vi "sub_UIupdate_rt.vi"(11 "log data":T1) -> (0 "error out":errorcluster)   [LabVIEW 2016]
uses:
  ctl/log_data.ctl
  ctl/UI_cmd-ctl.ctl
  <vilib>/Analysis/baseanly.llb/Mean (DBL).vi
  Global.vi
  <vilib>/Analysis/baseanly.llb/Unimode.vi
  <vilib>/Analysis/NI_AALBase.lvlib
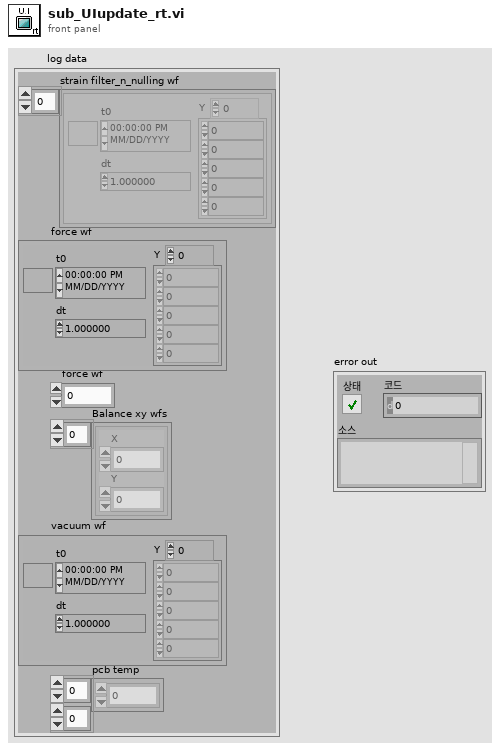
[diagram p1: front panel]
types:
  T1 = typedef "log_data.ctl" = cluster{"strain filter_n_nulling wf":waveform(dbl)[], "force wf":waveform(dbl), "force":dbl, "Balance xy wfs":cluster{"X":dbl, "Y":dbl}[], "vacuum kpa wf":waveform(dbl), "pcb temp":dbl[][]}
  T2 = typedef "UI_cmd-ctl.ctl" = enum16{"default", "create", "read"}
  T3 = typedef "UI_ctl.ctl" = cluster{"Heater temp":refnum<vi>, "Heater chart":refnum<vi>, "vacuum (kpa)":refnum<vi>, "Balance xy graph":refnum<vi>, "Strain chart w cal":refnum<vi>, "Pickup force":refnum<vi>, "Pickup time":refnum<vi>, "Force chart":refnum<vi>, "Force graph T":refnum<vi>, "vacuum chart":refnum<vi>, "vacuum rt":refnum<vi>, "Strain raw graph":refnum<vi>, "Strain raw chart":refnum<vi>, "Bonding time":refnum<vi>, "Bonding force":refnum<vi>, "Balance":refnum<vi>, "Filtered force graph":refnum<vi>, "ROI intensity":refnum<vi>, "Heater_rt":refnum<vi>, "Detach force":refnum<vi>, "Force rt":refnum<vi>, "Mixed signal":refnum<vi>}
  T4 = typedef "config_ctl.ctl" = cluster{"Lower Cut-Off":dbl, "Vacuum Trigger level":dbl, "state settings":cluster{"method":enum32{"histogram", "peak", "auto select"}, "histogram size":i32, "histogram method":enum16{"mode"}, "reserved":dbl}, "SPA-300 Setting":cluster{"Bonding force (g)":dbl, "Bonding time (ms)":dbl, "Pickup force (g)":dbl, "Pickup time (ms)":dbl, "Speed":enum16{"Slow", "Fast"}}, "sensor file":path}
  T5 = cluster{"PCB temp":refnum<vi>, "Vacuum":refnum<vi>, "PCB config":refnum<vi>, "Balance_x":refnum<vi>, "Balance_y":refnum<vi>}
  T6 = typedef "data.ctl" = cluster{"Bonding force":dbl, "Bonding time":dbl, "Bonding index":dbl, "Pickup force":dbl, "Pickup time":dbl, "Pickup index":dbl, "Detach force":dbl, "Detach time":dbl, "Detach index":dbl, "Heater temp rt":dbl, "Vacuum rt":dbl, "IR raw data":i16[][], "IR temp data":dbl[][], "vacuum raw wf":waveform(dbl), "vacuum kpa wf":waveform(dbl), "strain raw wf":waveform(dbl)[], "Force rt":dbl, "Vacuum T":dbl, "Heater temp T":dbl, "Balance xy arrays":cluster{dbl, dbl}[], "Balance xy":cluster{dbl, dbl}[], "Bonding wf index":dbl, "Pickup wf index":dbl, "Bonding rising index":dbl, "Bonding falling index":dbl, "Pickup rising index":dbl, "Pickup falling index":dbl}
  T7 = cluster{"Force rt":dbl, "Vacuum rt":dbl, "Heater temp rt":dbl}
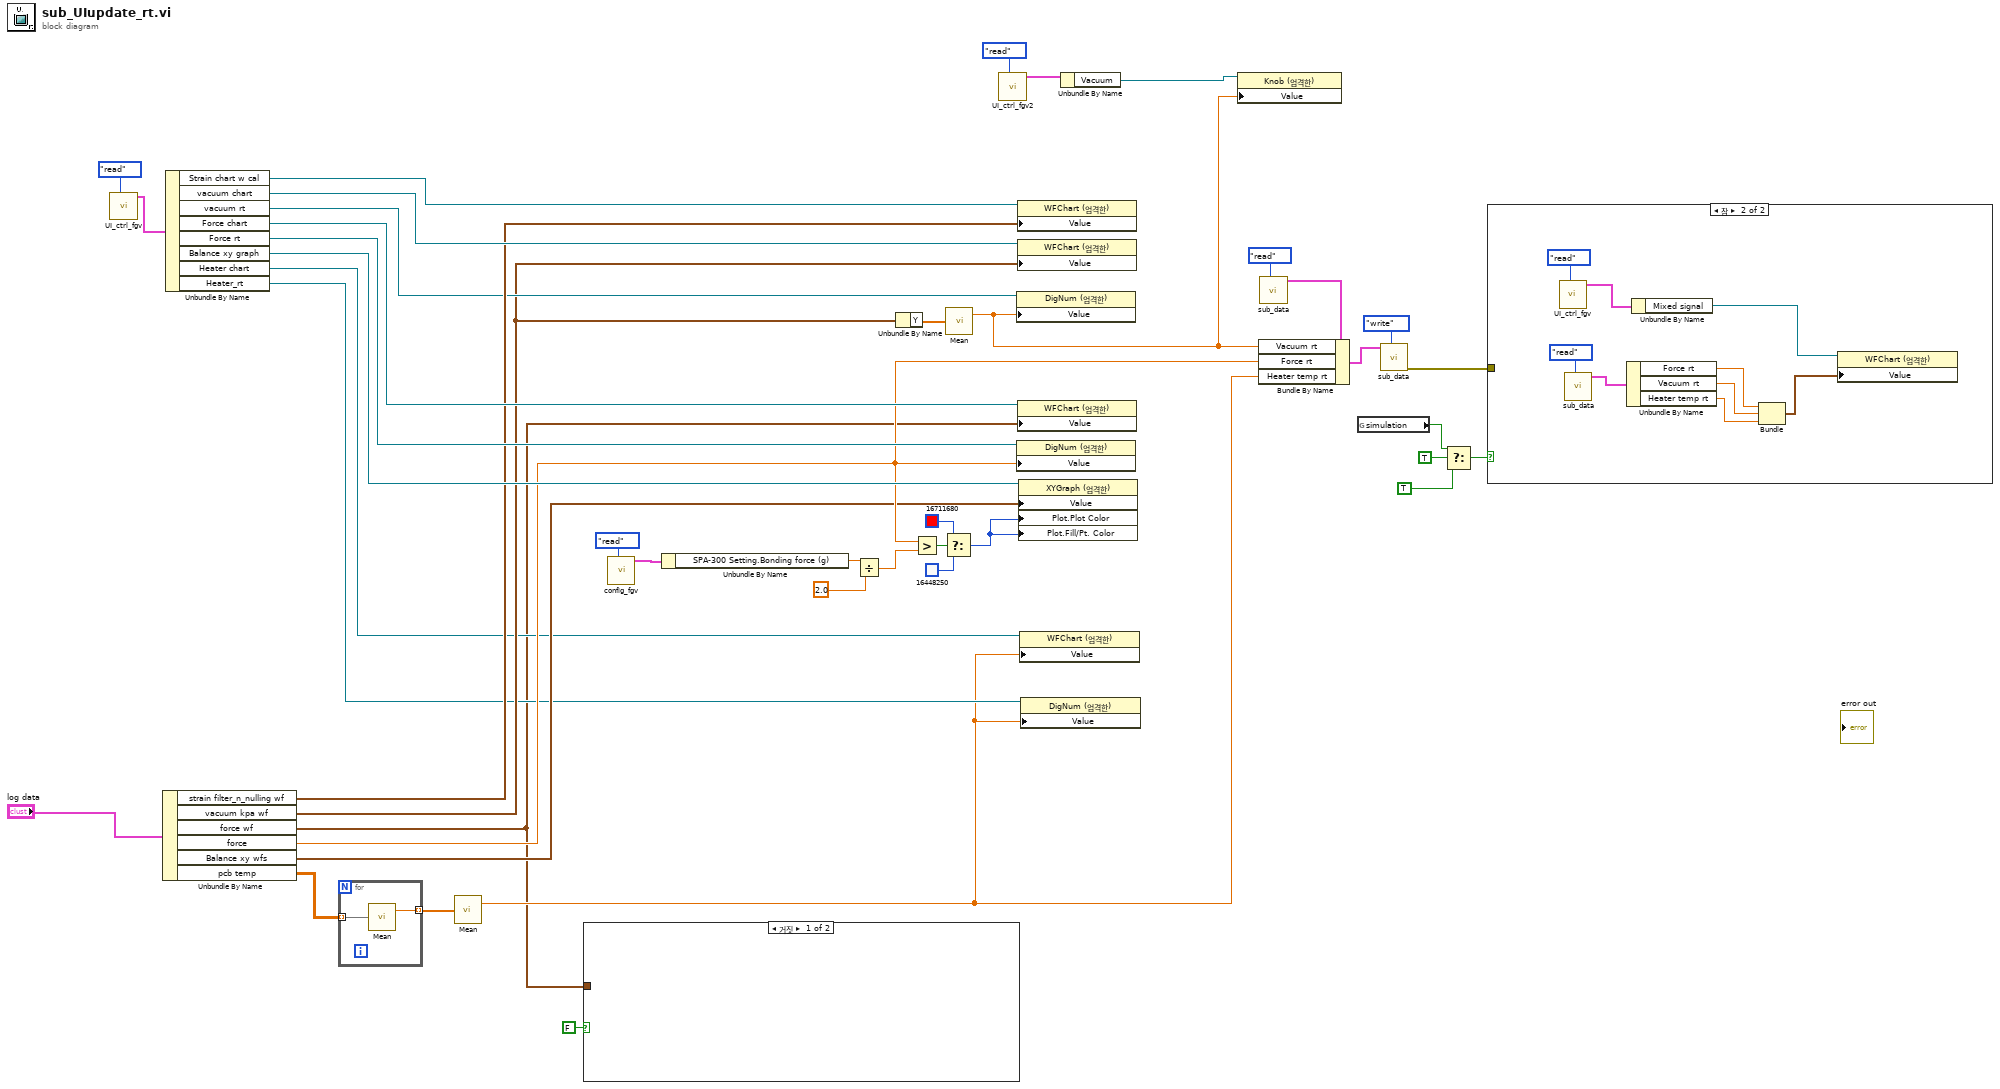
[diagram p0: block diagram]
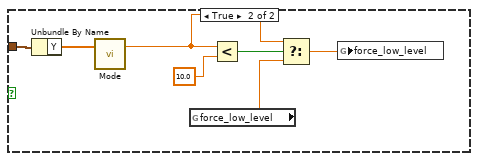
[diagram p2: hidden frame]
diagram:
  n1 = call "UI_ctrl_fgv.vi"("cmd"=UI_cmd-ctl."read") -> ("UI cluster out"=w39:T3)  [unwired: 10 in]
  n2 = Unbundle By Name("log data") -> ("strain filter_n_nulling wf"=w36:waveform(dbl)[], "vacuum kpa wf"=w31:waveform(dbl), "force wf"=w1:waveform(dbl), "force"=w19:dbl, "Balance xy wfs"=w14:cluster{"X":dbl, "Y":dbl}[], "pcb temp"=w18:dbl[][])
  n3 = Unbundle By Name(w39) -> ("Strain chart w cal"=w37:refnum<vi>, "vacuum chart"=w38:refnum<vi>, "vacuum rt"=w34:refnum<vi>, "Force chart"=w41:refnum<vi>, "Force rt"=w42:refnum<vi>, "Balance xy graph"=w43:refnum<vi>, "Heater chart"=w13:refnum<vi>, "Heater_rt"=w12:refnum<vi>)
  n4 = for {
    tunnel: w18 -> [w45] mode=indexing
    tunnel: [w44] -> w17 mode=indexing
    n5 = call-poly <vilib>:"Mean.vi"("X"=w45) -> ("mean"=w44:dbl)  [unwired: 1 out]
  }
  n6 = call-poly <vilib>:"Mean.vi"("X"=w17) -> ("mean"=w11:dbl)  [unwired: 1 out]
  n7 = case shown="거짓" FALSE {
    tunnel: w1 -> [_ w52]
    frame False {
    }
    frame True {
      n8 = Unbundle By Name(w52) -> ("Y"=w51:dbl[])
      n9 = call-poly <vilib>:"Mode.vi"("X"=w51) -> ("mode"=w48:dbl)  [unwired: 1 in, 1 out]
      n10 = global read "Global.vi" "force_low_level"() -> (w47:dbl)
      n11 = Less?(x=w48, y=10.0) -> (x < y?=w49:bool)
      n12 = Select(t=w48, s=w49, f=w47) -> (s? t:f=w46:dbl)
      n13 = global write "Global.vi" "force_low_level"(w46) -> ()
    }
  }
  n14 = call "config_fgv.vi"("cmd"=enum16{"write", "read", "ini"}."read") -> ("Config out"=w24:T4)  [unwired: 9 in, 1 out]
  n15 = Unbundle By Name(w24) -> ("SPA-300 Setting.Bonding force (g)"=w23:dbl)
  n16 = Divide(x=w23, y=2.0) -> (x/y=w21:dbl)
  n17 = Unbundle By Name(w31) -> ("Y"=w30:dbl[])
  n18 = Greater?(x=w19, y=w21) -> (0:w29:bool)
  n19 = Select(t=u32 16711680, s=w29, f=u32 16448250) -> (s? t:f=w26:u32)
  n20 = call-poly <vilib>:"Mean.vi"("X"=w30) -> ("mean"=w3:dbl)  [unwired: 1 out]
  n21 = call "UI_ctrl_fgv2.vi"("cmd"=enum16{"read", "create"}."read") -> ("UI out"=w5:T5)  [unwired: 10 in]
  n22 = property class="DigNum (엄격한)"(reference=w34, "Value"=w3) -> ()  [unwired: 1 in, 2 out]
  n23 = property class="DigNum (엄격한)"(reference=w42, "Value"=w19) -> ()  [unwired: 1 in, 2 out]
  n24 = property class="WFChart (엄격한)"(reference=w37, "Value"=w36) -> ()  [unwired: 1 in, 2 out]
  n25 = property class="WFChart (엄격한)"(reference=w38, "Value"=w31) -> ()  [unwired: 1 in, 2 out]
  n26 = property class="WFChart (엄격한)"(reference=w41, "Value"=w1) -> ()  [unwired: 1 in, 2 out]
  n27 = property class="XYGraph (엄격한)"(reference=w43, "Value"=w14, "Plot.Plot Color"=w26, "Plot.Fill/Pt. Color"=w26) -> ()  [unwired: 1 in, 2 out]
  n28 = property class="WFChart (엄격한)"(reference=w13, "Value"=w11) -> ()  [unwired: 1 in, 2 out]
  n29 = property class="DigNum (엄격한)"(reference=w12, "Value"=w11) -> ()  [unwired: 1 in, 2 out]
  n30 = Unbundle By Name(w5) -> ("Vacuum"=w4:refnum<vi>)
  n31 = property class="Knob (엄격한)"(reference=w4, "Value"=w3) -> ()  [unwired: 1 in, 2 out]
  n32 = call "sub_data.vi"("cmd"=enum16{"ini", "write", "read"}."read") -> ("data out"=w15:T6)  [unwired: 9 in, 1 out]
  n33 = Bundle By Name(cluster=w15, "Vacuum rt"=w3, "Force rt"=w19, "Heater temp rt"=w11) -> (w32:T6)
  n34 = global read "Global.vi" "simulation"() -> (w8:bool)
  n35 = call "sub_data.vi"("cmd"=enum16{"ini", "write", "read"}."write", "data in"=w32) -> ("error out"=w20:errorcluster)  [unwired: 8 in, 1 out]
  n36 = Select(t=w8, s=TRUE, f=TRUE) -> (s? t:f=w10:bool)
  n37 = case shown="참" w10 {
    tunnel: w20 -> [_ _]
    frame False {
    }
    frame True {
      n38 = call "UI_ctrl_fgv.vi"("cmd"=UI_cmd-ctl."read") -> ("UI cluster out"=w59:T3)  [unwired: 10 in]
      n39 = call "sub_data.vi"("cmd"=enum16{"ini", "write", "read"}."read") -> ("data out"=w57:T6)  [unwired: 9 in, 1 out]
      n40 = Unbundle By Name(w57) -> ("Force rt"=w56:dbl, "Vacuum rt"=w55:dbl, "Heater temp rt"=w53:dbl)
      n41 = Unbundle By Name(w59) -> ("Mixed signal"=w58:refnum<vi>)
      n42 = Bundle("Force rt"=w56, "Vacuum rt"=w55, "Heater temp rt"=w53) -> (w54:T7)  [unwired: 1 in]
      n43 = property class="WFChart (엄격한)"(reference=w58, "Value"=w54) -> ()  [unwired: 1 in, 2 out]
    }
  }
